vi "Grab Tag Information.vi"(8 "error in":errorcluster, 11 "VI Ref in":refnum<vi>) -> (0 "error out":errorcluster, 1 "Control Info":T1[](array[typedef]) {"Boolean Type" items=["N/A", "FAB--icon--rounded", "outline--icon--rectangular", "outline--icon--rounded", "outline--text--rectangular", "outline--text--rounded", "nooutline--icon--rectangular", "nooutline--icon--rectangular--40x40", "nooutline--icon--rounded", "nooutline--text--rectangular", "nooutline--text--rounded", "tonal--icon--rectangular", "tonal--icon--rounded", "tonal--text--rectangular", "tonal--text--rounded", "filled--icon--rectangular", "filled--icon--rounded", "filled--text--rectangular", "filled--text--rounded"]; "UI Theme Level" items=["N/A", "Primary", "Secondary", "Tertiary", "Error", "Primary Fixed", "Secondary Fixed", "Tertiary Fixed", "Label Only", "No Change"]}, 2 "map data":map{string, refnum<vi>}(c390), 3 "VI Ref out":refnum<vi>)   [LabVIEW 2021]
uses:
  control info.ctl
  <vilib>/Utility/traverseref.llb/TRef TravTarget.ctl
  <vilib>/Utility/traverseref.llb/VI Scripting - Traverse.lvlib
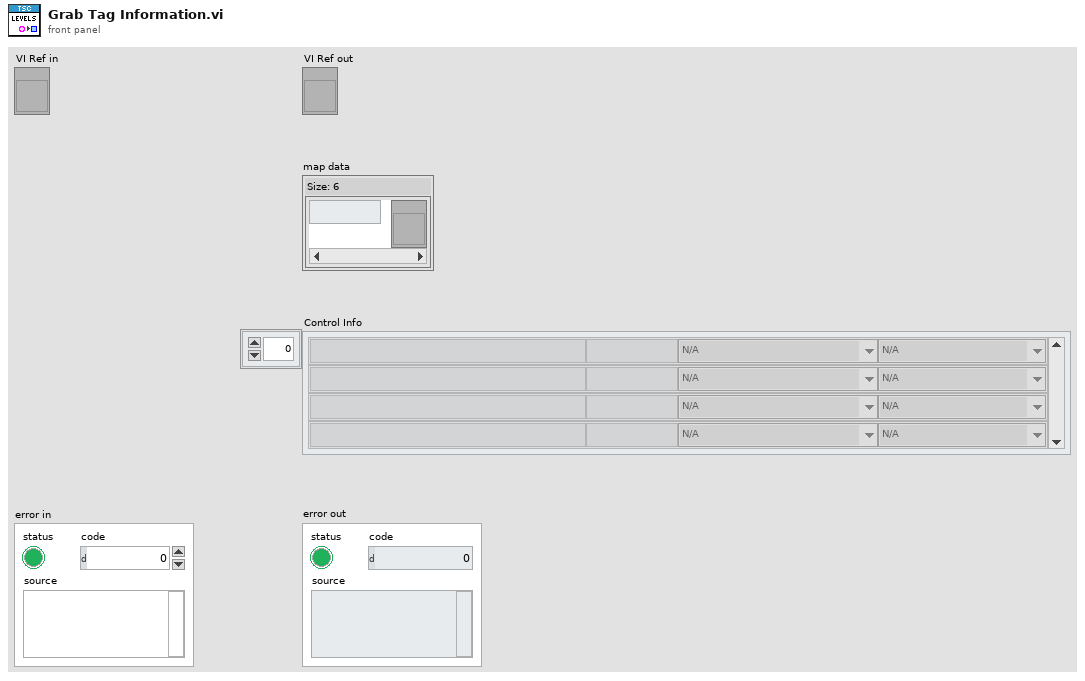
[diagram p1: front panel]
types:
  T1 = typedef "control info.ctl" = cluster{"label":string, "control type":string, "UI Theme Level":u16, "Boolean Type":u16}
  T2 = typedef "TRef TravTarget.ctl" = enum16{"FP", "BD", "Other"}
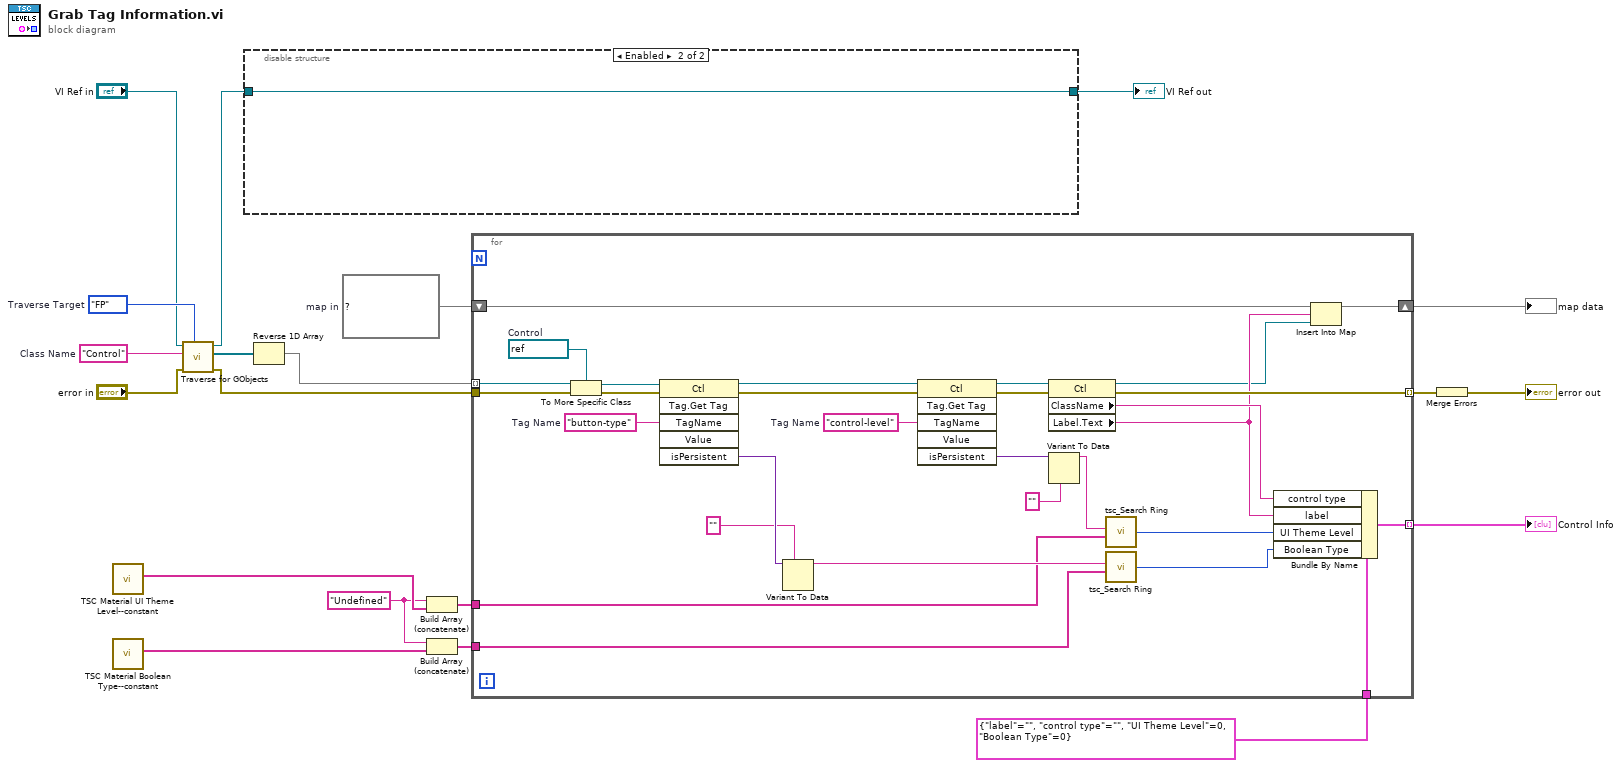
[diagram p0: block diagram]
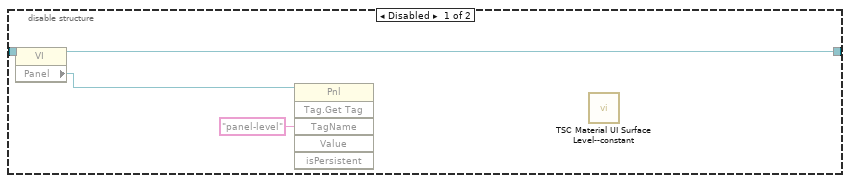
[diagram p2: hidden frame]
diagram:
  w7 = TRef_TravTarget."FP"  # Traverse Target
  w8 = "Control"  # Class Name
  w11 = "Undefined"
  w16 = map{string, refnum<vi>} {}  # map in
  n1 = call "TSC Material UI Theme Level--constant.vi"() -> ("UI theme levels"=w13:string[])  [unwired: 11 in]
  n2 = call "TSC Material Boolean Type--constant.vi"() -> ("boolean types"=w12:string[])  [unwired: 11 in]
  n3 = call <vilib>:"Traverse for GObjects.vi"("Traverse Target"=w7, "error in (no error)"="error in", "Class Name"=w8, "VI Refnum"="VI Ref in") -> ("error out"=w19:errorcluster, "References"=w6:refnum<vi>[], "dup VI Refnum"=w2:refnum<vi>)  [unwired: 4 in, 1 out]
  n4 = disable-structure shown="Enabled" {
    disable-tunnel: w2 -> [w23 w25]
    disable-tunnel: [w21 w25] -> w1
    frame Disabled {
      n5 = property class="VI"(reference=w23) -> (reference out=w21:refnum<vi>, "Panel"=w22:refnum<vi>)  [unwired: 1 in, 1 out]
      n6 = invoke class="Pnl" method="Tag.Get Tag"(reference=w22, "TagName"="panel-level" ("Tag Name")) -> ()  [unwired: 4 in, 6 out]
      n7 = call "TSC Material UI Surface Level--constant.vi"() -> ()  [unwired: 11 in, 1 out]
    }
    frame Enabled {
    }
  }
  "VI Ref out" <- w1
  n8 = Reverse 1D Array(array=w6) -> (reversed array=w4:refnum<vi>[])
  n9 = Build Array (concatenate)(w11, w13) -> (w10:string[])
  n10 = Build Array (concatenate)(w11, w12) -> (w9:string[])
  n11 = for {
    tunnel: w4 -> [w41] mode=indexing
    tunnel: w19 -> [w54]
    tunnel: [w51] -> w3 mode=indexing
    tunnel: T1 {"label"="", "control type"="", "UI Theme Level"=0, "Boolean Type"=0} ("control info") -> [w38]
    tunnel: [w36] -> w15 mode=indexing
    shift-right: [w34] -> w17
    shift-left: w16 -> [w35]
    tunnel: w10 -> [w27]
    tunnel: w9 -> [w26]
    w39 = refnum<vi> refnum  # Control
    w43 = "control-level"  # Tag Name
    w49 = "button-type"  # Tag Name
    n12 = To More Specific Class(target class=w39, reference=w41, error in=w54) -> (specific class reference=w40:refnum<vi>, error out=w50:errorcluster)
    n13 = invoke class="Ctl" method="Tag.Get Tag"(reference=w40, error in=w50, "TagName"=w49) -> (reference out=w46:refnum<vi>, error out=w53:errorcluster, "isPersistent"=w48:variant)  [unwired: 3 in, 3 out]
    n14 = Variant To Data(type="", Variant=w48) -> (data=w29:string)  [unwired: 1 in, 1 out]
    n15 = invoke class="Ctl" method="Tag.Get Tag"(reference=w46, error in=w53, "TagName"=w43) -> (reference out=w42:refnum<vi>, error out=w52:errorcluster, "isPersistent"=w44:variant)  [unwired: 3 in, 3 out]
    n16 = property class="Ctl"(reference=w42, error in=w52) -> (reference out=w32:refnum<vi>, error out=w51:errorcluster, "ClassName"=w37:string, "Label.Text"=w33:string)
    n17 = Variant To Data(type="", Variant=w44) -> (data=w31:string)  [unwired: 1 in, 1 out]
    n18 = call "tsc_Search Ring.vi"("Values"=w27, "Search Item"=w31) -> ("Index"=w30:u16)  [unwired: 2 in]
    n19 = call "tsc_Search Ring.vi"("Values"=w26, "Search Item"=w29) -> ("Index"=w28:u16)  [unwired: 2 in]
    n20 = Bundle By Name(cluster=w38, "control type"=w37, "label"=w33, "UI Theme Level"=w30, "Boolean Type"=w28) -> (w36:T1)
    n21 = Insert Into Map(map in=w35, key=w33, value=w32) -> (map out=w34:map{string, refnum<vi>})  [unwired: 2 out]
  }
  "map data" <- w17
  "Control Info" <- w15
  n22 = Merge Errors(w3) -> (→"error out":errorcluster)
